vi "Get Enqueuer.vi"(8 "error in":errorcluster, 10 "Ex Nested":refnum<class "Ex Nested.lvclass">=refnum, 11 "Controller in":refnum<class "Controller.lvclass">) -> (0 "error out":errorcluster, 2 "Enqueuer":refnum<class "Message Enqueuer.lvclass">, 3 "Controller out":refnum<class "Controller.lvclass">)   [LabVIEW 2014, in "Controller.lvlib" / "Controller.lvclass"]
uses:
  Controller.lvclass
  <vilib>/ActorFramework/Message Enqueuer/Message Enqueuer.lvclass
  Controls/eMap.ctl
  SuperActor/Ex Nested.lvclass
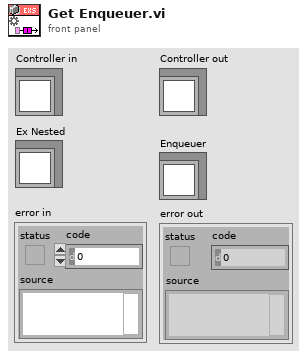
[diagram p1: front panel]
types:
  T1 = typedef "Controller.lvlib/Controller.lvclass/eMap.ctl" = cluster{"Enqueuer":refnum<class "Message Enqueuer.lvclass">, "Active":bool}
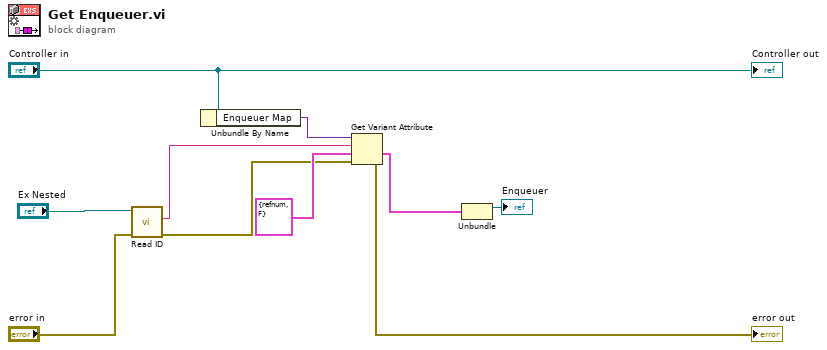
[diagram p0: block diagram]
diagram:
  n1 = call "Read ID.vi"("error in (no error)"="error in", "Ex Nested in"="Ex Nested") -> ("error out"=w3:errorcluster, "ID"=w6:string)  [unwired: 7 in, 1 out]
  n2 = Unbundle By Name("Controller in") -> ("Enqueuer Map"=w9:variant)
  n3 = Get Variant Attribute(Variant=w9, name=w6, default value (empty Variant)=T1 {"Enqueuer"=refnum, "Active"=FALSE} ("eMap"), error in=w3) -> (value=w5:T1, error out=→"error out":errorcluster)  [unwired: 2 out]
  n4 = Unbundle(w5) -> ("Enqueuer"=→"Enqueuer":refnum<class "Message Enqueuer.lvclass">)  [unwired: 1 out]
  "Controller out" <- "Controller in"
